vi "Read SS2 Data Information.vi"(8 "error in (no error)":errorcluster, 11 "group in":T2 format="%.0x") -> (0 "error out":errorcluster, 2 "Data Information":T1, 3 "group out":T2 format="%.0x")   [LabVIEW 2021, in "SwissSPAD.lvlib"]
uses:
  SwissSPAD.lvlib
  <vilib>/addons/h5labview2/base/hid_t.ctl
  SS2 Data Information.ctl
  SS2 Data Information List.ctl
  <vilib>/addons/h5labview2/base/lib_path.vi
  <vilib>/addons/h5labview2/base/H5Equery.vi
  <vilib>/addons/h5labview2/dataset/H5Dread.llb/H5Dread.xnode
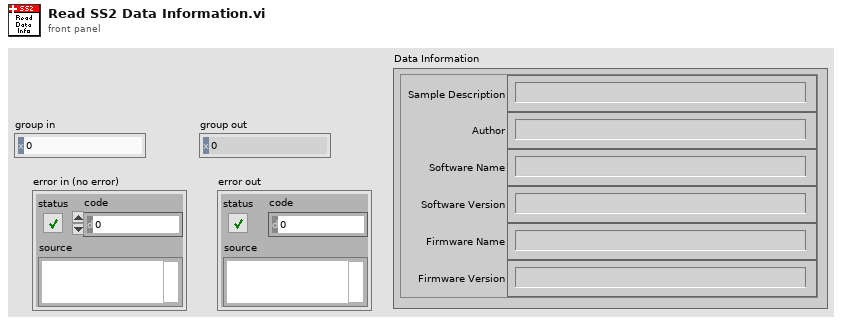
[diagram p1: front panel]
types:
  T1 = typedef "SwissSPAD.lvlib/SS2 Data Information.ctl" = cluster{"Sample Description":string, "Author":string, "Software Name":string, "Software Version":string, "Firmware Name":string, "Firmware Version":string}
  T2 = typedef "hid_t.ctl" = i64
  T3 = typedef "SwissSPAD.lvlib/SS2 Data Information List.ctl" = enum16{"author", "description", "software_name", "software_version", "firmware_name", "firmware_version"}
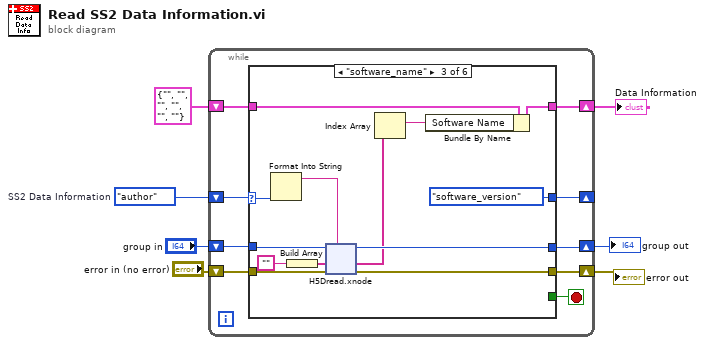
[diagram p0: block diagram]
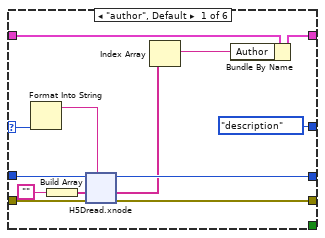
[diagram p2: hidden frame]
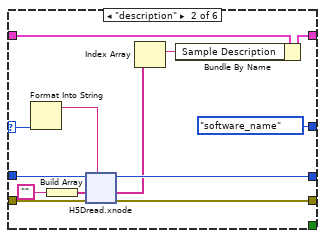
[diagram p3: hidden frame]
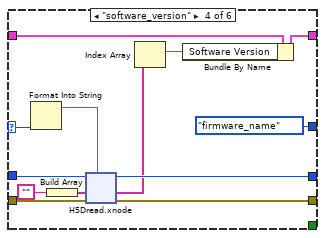
[diagram p4: hidden frame]
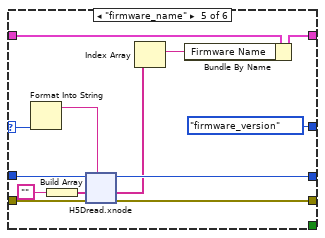
[diagram p5: hidden frame]
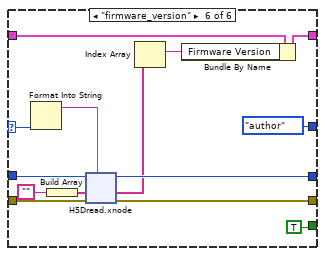
[diagram p6: hidden frame]
diagram:
  w3 = SS2_Data_Information_List."author"  # SS2 Data Information
  n1 = while {
    shift-right: [w10] -> w1
    shift-left: T1 {"Sample Description"="", "Author"="", "Software Name"="", "Software Version"="", "Firmware Name"="", "Firmware Version"=""} ("Data Information") -> [w11]
    shift-right: [w12] -> w6
    shift-left: "error in (no error)" -> [w13]
    shift-right: [w14] -> w4
    shift-left: "group in" -> [w15]
    shift-right: [w9] -> _
    shift-left: w3 -> [w16]
    stop <- w8 stop-if-true
    n2 = case shown="\"software_name\"" w16 {
      selector: w16 -> [w28 w56 w84 w112 w140 w169]
      tunnel: w15 -> [w27 w55 w83 w111 w139 w168]
      tunnel: [w26 w54 w82 w110 w138 w167] -> w14
      tunnel: w13 -> [w25 w53 w81 w109 w137 w166]
      tunnel: [w24 w52 w80 w108 w136 w165] -> w12
      tunnel: w11 -> [w22 w50 w78 w106 w134 w163]
      tunnel: [w20 w48 w76 w104 w132 w161] -> w10
      tunnel: [SS2_Data_Information_List."description" ("SS2 Data Information") SS2_Data_Information_List."software_name" ("SS2 Data Information") SS2_Data_Information_List."software_version" ("SS2 Data Information") SS2_Data_Information_List."firmware_name" ("SS2 Data Information") SS2_Data_Information_List."firmware_version" ("SS2 Data Information") SS2_Data_Information_List."author" ("SS2 Data Information")] -> w9
      tunnel: [_ _ _ _ _ TRUE] -> w8
      frame "author", Default {
        n3 = Format Into String(w28) -> (resulting string=w29:string)  [unwired: 3 in, 1 out]
        n4 = Build Array("") -> (w19:string[])
        n5 = xnode "H5Dread.xnode"("dataset name (this)"=w29, "error in (no error)"=w25, "default"=w19, "ref in"=w27) -> ("error out"=w24:errorcluster, "data"=w21:string[], "ref out"=w26:T2)  [unwired: 2 in, 1 out]
        n6 = Index Array(array=w21) -> (element=w17:string)  [unwired: 1 in]
        n7 = Bundle By Name(cluster=w22, "Author"=w17) -> (w20:T1)
      }
      frame "description" {
        n8 = Format Into String(w56) -> (resulting string=w57:string)  [unwired: 3 in, 1 out]
        n9 = Build Array("") -> (w47:string[])
        n10 = xnode "H5Dread.xnode"("dataset name (this)"=w57, "error in (no error)"=w53, "default"=w47, "ref in"=w55) -> ("error out"=w52:errorcluster, "data"=w49:string[], "ref out"=w54:T2)  [unwired: 2 in, 1 out]
        n11 = Index Array(array=w49) -> (element=w45:string)  [unwired: 1 in]
        n12 = Bundle By Name(cluster=w50, "Sample Description"=w45) -> (w48:T1)
      }
      frame "software_name" {
        n13 = Format Into String(w84) -> (resulting string=w85:string)  [unwired: 3 in, 1 out]
        n14 = Build Array("") -> (w75:string[])
        n15 = xnode "H5Dread.xnode"("dataset name (this)"=w85, "error in (no error)"=w81, "default"=w75, "ref in"=w83) -> ("error out"=w80:errorcluster, "data"=w77:string[], "ref out"=w82:T2)  [unwired: 2 in, 1 out]
        n16 = Index Array(array=w77) -> (element=w73:string)  [unwired: 1 in]
        n17 = Bundle By Name(cluster=w78, "Software Name"=w73) -> (w76:T1)
      }
      frame "software_version" {
        n18 = Format Into String(w112) -> (resulting string=w113:string)  [unwired: 3 in, 1 out]
        n19 = Build Array("") -> (w103:string[])
        n20 = xnode "H5Dread.xnode"("dataset name (this)"=w113, "error in (no error)"=w109, "default"=w103, "ref in"=w111) -> ("error out"=w108:errorcluster, "data"=w105:string[], "ref out"=w110:T2)  [unwired: 2 in, 1 out]
        n21 = Index Array(array=w105) -> (element=w101:string)  [unwired: 1 in]
        n22 = Bundle By Name(cluster=w106, "Software Version"=w101) -> (w104:T1)
      }
      frame "firmware_name" {
        n23 = Format Into String(w140) -> (resulting string=w141:string)  [unwired: 3 in, 1 out]
        n24 = Build Array("") -> (w131:string[])
        n25 = xnode "H5Dread.xnode"("dataset name (this)"=w141, "error in (no error)"=w137, "default"=w131, "ref in"=w139) -> ("error out"=w136:errorcluster, "data"=w133:string[], "ref out"=w138:T2)  [unwired: 2 in, 1 out]
        n26 = Index Array(array=w133) -> (element=w129:string)  [unwired: 1 in]
        n27 = Bundle By Name(cluster=w134, "Firmware Name"=w129) -> (w132:T1)
      }
      frame "firmware_version" {
        n28 = Format Into String(w169) -> (resulting string=w170:string)  [unwired: 3 in, 1 out]
        n29 = Build Array("") -> (w160:string[])
        n30 = xnode "H5Dread.xnode"("dataset name (this)"=w170, "error in (no error)"=w166, "default"=w160, "ref in"=w168) -> ("error out"=w165:errorcluster, "data"=w162:string[], "ref out"=w167:T2)  [unwired: 2 in, 1 out]
        n31 = Index Array(array=w162) -> (element=w158:string)  [unwired: 1 in]
        n32 = Bundle By Name(cluster=w163, "Firmware Version"=w158) -> (w161:T1)
      }
    }
  }
  "group out" <- w4
  "error out" <- w6
  "Data Information" <- w1
